vi "Commit NVMEM (Core).vi"(7 "nvmem type":T1, 8 "error in (no error)":errorcluster, 10 "resources":string, 11 "SLSC Local in":refnum<class "SLSC Local.lvclass">) -> (0 "error out":errorcluster, 3 "SLSC Local out":refnum<class "SLSC Local.lvclass">)   [LabVIEW 2015, in "SLSC Local.lvclass"]
uses:
  SLSC Local.lvclass
  <vilib>/SLSC/SLSC.lvlib
  <vilib>/SLSC/Commit NVMEM for Devices.vi
  <vilib>/SLSC/Commit NVMEM for Session.vi
  <vilib>/SLSC/Commit NVMEM Areas.vi
  SLSC Interface Class/nvmem type.ctl
  SLSC Interface Class/SLSC Interface.lvclass
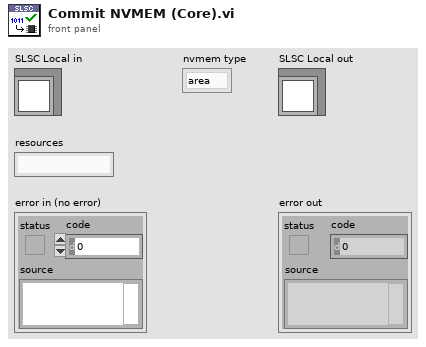
[diagram p1: front panel]
types:
  T1 = typedef "SLSC Interface.lvclass/nvmem type.ctl" = enum16{"area", "device", "session"}
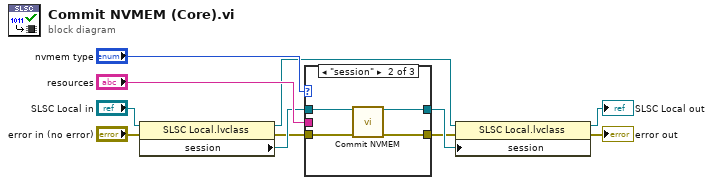
[diagram p0: block diagram]
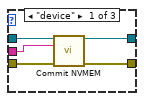
[diagram p2: hidden frame]
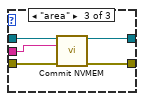
[diagram p3: hidden frame]
diagram:
  n1 = property class="SLSC Local.lvclass"(reference="SLSC Local in", error in="error in (no error)") -> (reference out=w7:refnum<class "SLSC Local.lvclass">, error out=w3:errorcluster, "session"=w9:refnum<k21>)
  n2 = case shown="\"session\"" "nvmem type" {
    tunnel: "resources" -> [w16 _ w21]
    tunnel: w9 -> [w15 w20 w25]
    tunnel: [w14 w19 w24] -> w5
    tunnel: w3 -> [w13 w18 w23]
    tunnel: [w12 w17 w22] -> w2
    frame "device" {
      n3 = call-poly <vilib>:"Commit NVMEM.vi"("session in"=w15, "devices"=w16, "error in (no error)"=w13) -> ("session out"=w14:refnum<k21>, "error out"=w12:errorcluster)  [unwired: 11 in]
    }
    frame "session" {
      n4 = call-poly <vilib>:"Commit NVMEM.vi"("session in"=w20, "error in (no error)"=w18) -> ("session out"=w19:refnum<k21>, "error out"=w17:errorcluster)  [unwired: 12 in]
    }
    frame "area" {
      n5 = call-poly <vilib>:"Commit NVMEM.vi"("session in"=w25, "NVMEM areas"=w21, "error in (no error)"=w23) -> ("session out"=w24:refnum<k21>, "error out"=w22:errorcluster)  [unwired: 11 in]
    }
  }
  n6 = property class="SLSC Local.lvclass"(reference=w7, error in=w2, "session"=w5) -> (reference out=→"SLSC Local out":refnum<class "SLSC Local.lvclass">, error out=→"error out":errorcluster)
